vi "Engine - Copy & Script Templates.vi"(7 "CD Name":string, 8 "error in (no error)":errorcluster, 9 "RT Driver VI Path":path, 10 "RT Driver Folder Path":path, 11 "CD Source Folder Path":path) -> (0 "error out":errorcluster)   [LabVIEW 2015, in "NIVS_Consolidated_CDW_MetaDataObj.lvclass"]
doc: "Via scripting, replace the tempate RTStateVariables control with the new type def across the async and RT driver VIs, and script the compiled settings property into the constants global"
uses:
  NIVS_Consolidated_CDW_MetaDataObj.lvclass
  Common.ctl
  <vilib>/Utility/traverseref.llb/TRef TravTarget.ctl
  CD Engine lvlib.ctl
  CD Shared lvlib.ctl
  Common.vi
  CD Engine lvlib.vi
  CD Shared lvlib.vi
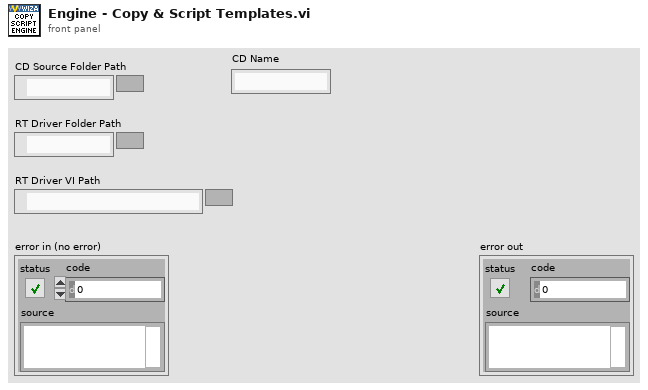
[diagram p1: front panel]
types:
  T1 = typedef "NIVS_Consolidated_CDW_MetaDataObj.lvclass/CD Engine lvlib.ctl" = enum16{"LibraryFileName", "LibraryFolderName", "Engine.FolderName", "Engine.Init.FolderName", "Engine.Run.FolderName", "Engine.Shutdown.FolderName", "Types.FolderName", "Engine.RT Driver VI.TemplatePath", "Engine.RT Driver VI.FileName", "Engine.RTStateVariables.Name", "Engine.RTStateVariables.Name.NoExtension", "Engine.Async.NameExtension", "Engine.Async.TemplateName"}
  T2 = typedef "NIVS_Consolidated_CDW_MetaDataObj.lvclass/CD Shared lvlib.ctl" = enum16{"LibraryFileName", "LibraryFolderName", "ConstantsVI.VIPathAndName", "Shared.FolderName", "Shared.Types.FolderName", "Shared.Constants.VIName", "Shared.Constants.VITemplateName", "Shared.Constants.VITemplatePathAndName", "Shared.CompiledSettings.RelativePath", "Shared.Constants.RelativePath", "Shared.CompiledSettings.Name", "Shared.CompiledSettings.Name.NoExtension", "Shared.CompiledSettings.ClusterName"}
  T3 = typedef "TRef TravTarget.ctl" = enum16{"FP", "BD", "Other"}
  T4 = typedef "NIVS_Consolidated_CDW_MetaDataObj.lvclass/Common.ctl" = enum16{"ProjectName", "TemplatesFolderName", "ProjectTemplatePathAndName", "TimingAndSyncFolderName", "CustomDeviceFolderName", "PathToTemplates"}
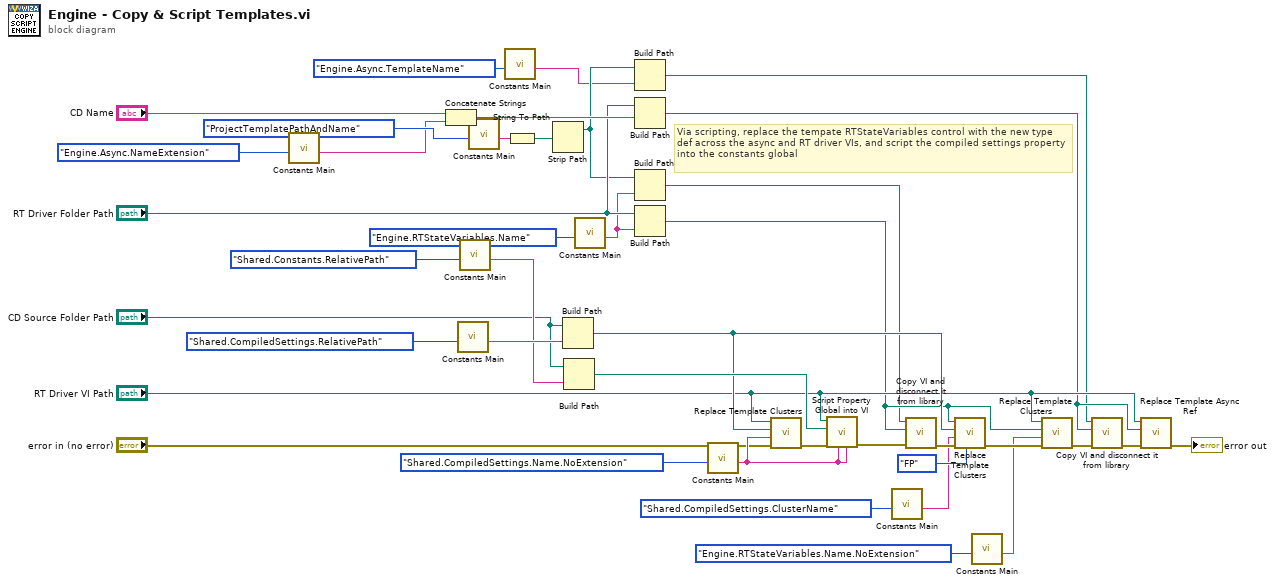
[diagram p0: block diagram]
diagram:
  # "Via scripting, replace the tempate RTStateVariables control with the new type def across the async and RT driver VIs, and script the compiled settings property into the constants global"
  n1 = call-poly "Constants Main.vi"("Action"=CD_Engine_lvlib."Engine.Async.NameExtension") -> ("Output"=w18:string)  [unwired: 10 in]
  n2 = Concatenate Strings("CD Name", w18) -> (w32:string)
  n3 = call-poly "Constants Main.vi"("Action"=CD_Shared_lvlib."Shared.CompiledSettings.RelativePath") -> ("Output"=w14:string)  [unwired: 10 in]
  n4 = call-poly "Constants Main.vi"("Action"=CD_Shared_lvlib."Shared.Constants.RelativePath") -> ("Output"=w12:string)  [unwired: 10 in]
  n5 = call-poly "Constants Main.vi"("Action"=Common."ProjectTemplatePathAndName") -> ("Output"=w21:string)  [unwired: 10 in]
  n6 = call-poly "Constants Main.vi"("Action"=CD_Engine_lvlib."Engine.Async.TemplateName") -> ("Output"=w16:string)  [unwired: 10 in]
  n7 = String To Path(string=w21) -> (path=w22:path)
  n8 = Strip Path(path=w22) -> (stripped path=w28:path)  [unwired: 1 out]
  n9 = Build Path(base path="CD Source Folder Path", name or relative path=w14) -> (appended path=w39:path)
  n10 = Build Path(base path="CD Source Folder Path", name or relative path=w12) -> (appended path=w40:path)
  n11 = call-poly "Constants Main.vi"("Action"=CD_Engine_lvlib."Engine.RTStateVariables.Name") -> ("Output"=w9:string)  [unwired: 10 in]
  n12 = Build Path(base path=w28, name or relative path=w16) -> (appended path=w31:path)
  n13 = Build Path(base path="RT Driver Folder Path", name or relative path=w32) -> (appended path=w35:path)
  n14 = Build Path(base path=w28, name or relative path=w9) -> (appended path=w23:path)
  n15 = Build Path(base path="RT Driver Folder Path", name or relative path=w9) -> (appended path=w27:path)
  n16 = call-poly "Constants Main.vi"("Action"=CD_Shared_lvlib."Shared.CompiledSettings.Name.NoExtension") -> ("Output"=w7:string)  [unwired: 10 in]
  n17 = call "Replace Template Clusters.vi"("error in (no error)"="error in (no error)", "Control Name"=w7, "Path to Cluster to Replace"=w39, "Path to VI"="RT Driver VI Path") -> ("error out"=w36:errorcluster)  [unwired: 7 in]
  n18 = call "Script Property Global into VI.vi"("GlobalControlName"=w7, "StringConstantToReplace"=w7, "error in (no error)"=w36, "Path to Global"=w40, "Path to VI"="RT Driver VI Path") -> ("error out"=w37:errorcluster)  [unwired: 6 in]
  n19 = call-poly "Constants Main.vi"("Action"=CD_Shared_lvlib."Shared.CompiledSettings.ClusterName") -> ("Output"=w5:string)  [unwired: 10 in]
  n20 = call "Copy VI and disconnect it from library.vi"("error in (no error)"=w37, "VI Target Path"=w27, "VI Source Path"=w23) -> ("error out"=w24:errorcluster)  [unwired: 8 in]
  n21 = call "Replace Template Clusters.vi"("Traverse Target"=TRef_TravTarget."FP", "error in (no error)"=w24, "Control Name"=w5, "Path to Cluster to Replace"=w39, "Path to VI"=w27) -> ("error out"=w26:errorcluster)  [unwired: 6 in]
  n22 = call-poly "Constants Main.vi"("Action"=CD_Engine_lvlib."Engine.RTStateVariables.Name.NoExtension") -> ("Output"=w3:string)  [unwired: 10 in]
  n23 = call "Replace Template Clusters.vi"("error in (no error)"=w26, "Control Name"=w3, "Path to Cluster to Replace"=w27, "Path to VI"="RT Driver VI Path") -> ("error out"=w30:errorcluster)  [unwired: 7 in]
  n24 = call "Copy VI and disconnect it from library.vi"("error in (no error)"=w30, "VI Target Path"=w35, "VI Source Path"=w31) -> ("error out"=w33:errorcluster)  [unwired: 8 in]
  n25 = call "Replace Template Async Ref.vi"("error in (no error)"=w33, "Path to Desired Async VI"=w35, "Path to RT Driver VI"="RT Driver VI Path") -> ("error out"=→"error out":errorcluster)  [unwired: 8 in]
